vi "Fetch Measurement (DANL Floor).vi"(8 "error in (no error)":errorcluster, 11 "VISA resource name":refnum<visa-resource-name>) -> (0 "error out":errorcluster, 3 "VISA resource name out":refnum<visa-resource-name>)   [LabVIEW 2014, in "Agilent ESA PSA Series.lvlib"]
doc: "Saves and reloads the DANL traces after taking a DANL Floor measurement.\n\n<B>Note:</B> \n\nThis VI is only valid for the Log Plot functionality of the Phase noise personality."
uses:
  Agilent ESA PSA Series.lvlib
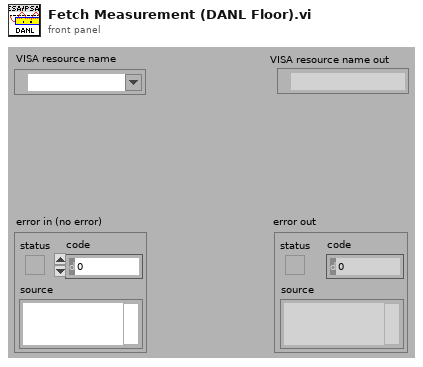
[diagram p1: front panel]
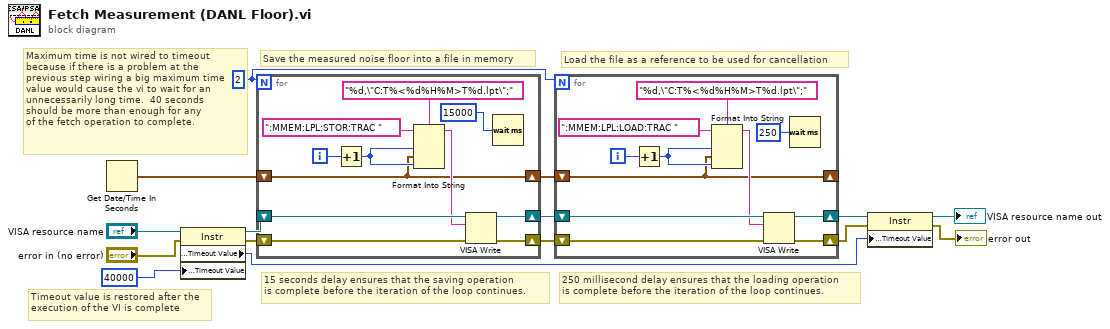
[diagram p0: block diagram]
diagram:
  w4 = 2
  # "Maximum time is not wired to timeout\nbecause if there is a problem at the\nprevious step wiring a big maximum time\nvalue would cause the vi to wait for an\nunnecessarily long time.  40 seconds\nshould be more than enough for any\nof the fetch operation to complete."
  # "250 millisecond delay ensures that the loading operation\nis complete before the iteration of the loop continues."
  # "15 seconds delay ensures that the saving operation\nis complete before the iteration of the loop continues."
  # "Timeout value is restored after the\nexecution of the VI is complete"
  # "Load the file as a reference to be used for cancellation"
  # "Save the measured noise floor into a file in memory"
  n1 = Get Date/Time In Seconds() -> (seconds since 1Jan1904=w8:timestamp)
  n2 = property on="Property Node" class="Instr"(reference="VISA resource name", error in="error in (no error)", "General Settings:Timeout Value"=u32 40000) -> (reference out=w10:refnum<visa-resource-name>, error out=w9:errorcluster, "General Settings:Timeout Value"=w13:u32)
  n3 = for {
    N: w4 -> [_]
    shift-right: [w23] -> w6
    shift-left: w10 -> [w25]
    shift-right: [w22] -> w5
    shift-left: w9 -> [w24]
    shift-right: [w17] -> w7
    shift-left: w8 -> [w17]
    i -> [w26]
    n4 = Increment(x=w26) -> (x+1=w18:i32)
    n5 = Format Into String(format string="%d,\"C:T%<%d%H%M>T%d.lpt\";", initial string=":MMEM:LPL:STOR:TRAC ", w18, w17, w18) -> (resulting string=w19:string)  [unwired: 1 in, 1 out]
    n6 = VISA Write(VISA resource name=w25, write buffer=w19, error in (no error)=w24) -> (VISA resource name out=w23:refnum<visa-resource-name>, error out=w22:errorcluster)  [unwired: 1 out]
    n7 = Wait (ms)(milliseconds to wait=u32 15000) -> ()  [unwired: 1 out]
  }
  n8 = for {
    N: w4 -> [_]
    shift-right: [w34] -> w3
    shift-left: w6 -> [w36]
    shift-right: [w33] -> w2
    shift-left: w5 -> [w35]
    shift-right: [w28] -> _
    shift-left: w7 -> [w28]
    i -> [w37]
    n9 = Increment(x=w37) -> (x+1=w29:i32)
    n10 = Format Into String(format string="%d,\"C:T%<%d%H%M>T%d.lpt\";", initial string=":MMEM:LPL:LOAD:TRAC ", w29, w28, w29) -> (resulting string=w30:string)  [unwired: 1 in, 1 out]
    n11 = VISA Write(VISA resource name=w36, write buffer=w30, error in (no error)=w35) -> (VISA resource name out=w34:refnum<visa-resource-name>, error out=w33:errorcluster)  [unwired: 1 out]
    n12 = Wait (ms)(milliseconds to wait=u32 250) -> ()  [unwired: 1 out]
  }
  n13 = property on="Property Node" class="Instr"(reference=w3, error in=w2, "General Settings:Timeout Value"=w13) -> (reference out=→"VISA resource name out":refnum<visa-resource-name>, error out=→"error out":errorcluster)
